vi "Read logFileRefnum.vi"(11 "Log in":refnum<class "Log.lvclass">) -> (2 "logFileRefnum":refnum<file>, 3 "Log out":refnum<class "Log.lvclass">)   [LabVIEW 2015, in "Log.lvlib" / "Log.lvclass"]
uses:
  <userlib>/Common/Log/Log/Log.lvclass
  <userlib>/Common/Log/Log/Log.lvclass/Log.ctl
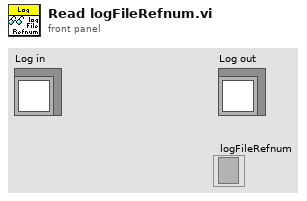
[diagram p1: front panel]
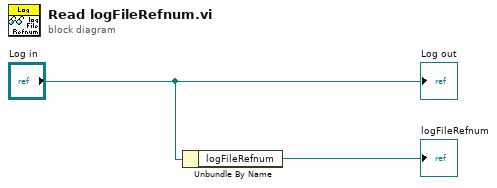
[diagram p0: block diagram]
diagram:
  n1 = Unbundle By Name("Log in") -> ("logFileRefnum"=→"logFileRefnum":refnum<file>)
  "Log out" <- "Log in"
